vi "Parse Sentence_VTG.vi"(8 "error in (no error)":errorcluster, 11 "VTG sentence":string) -> (0 "error out":errorcluster, 3 "VTG  data":T1 {"type of fix"."mode" items=["Simulator", "Not Valid", "Estimated", "Differential", "Autonomous"]})   [LabVIEW 2024]
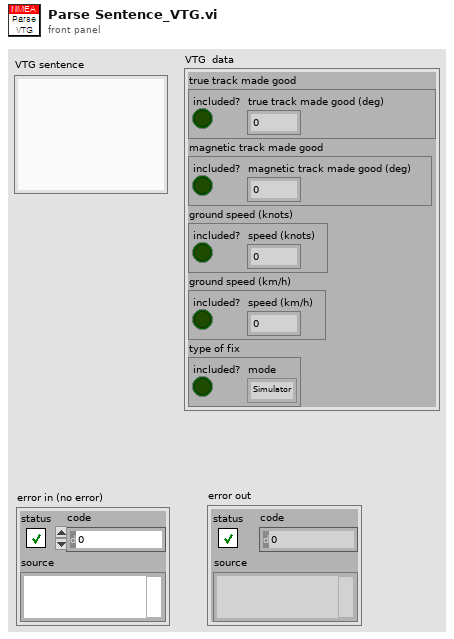
[diagram p1: front panel]
types:
  T1 = cluster{"true track made good":cluster{"included?":bool, "true track made good (deg)":dbl}, "magnetic track made good":cluster{"included?":bool, "magnetic track made good (deg)":dbl}, "ground speed (knots)":cluster{"included?":bool, "speed (knots)":dbl}, "ground speed (km/h)":cluster{"included?":bool, "speed (km/h)":dbl}, "type of fix":cluster{"included?":bool, "mode":u16}}
  T2 = cluster{"Boolean":bool, "True Track Made Good (Deg)":dbl}
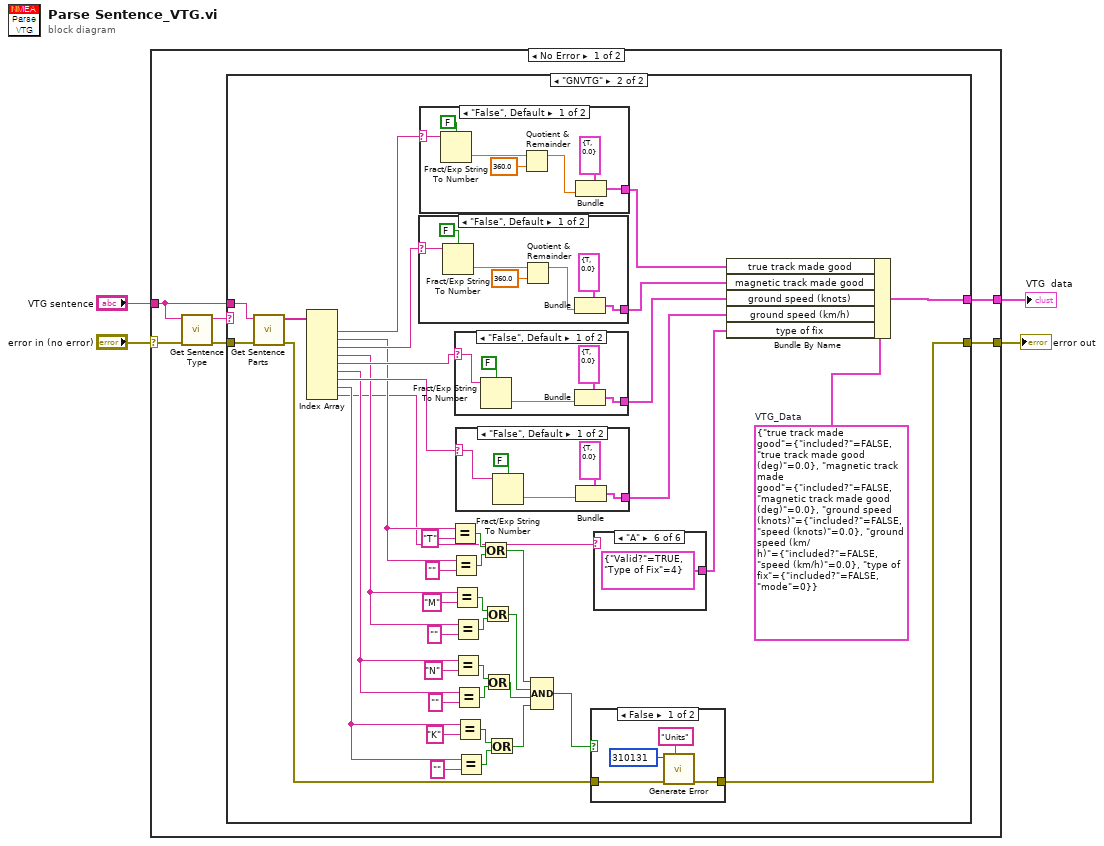
[diagram p0: block diagram]
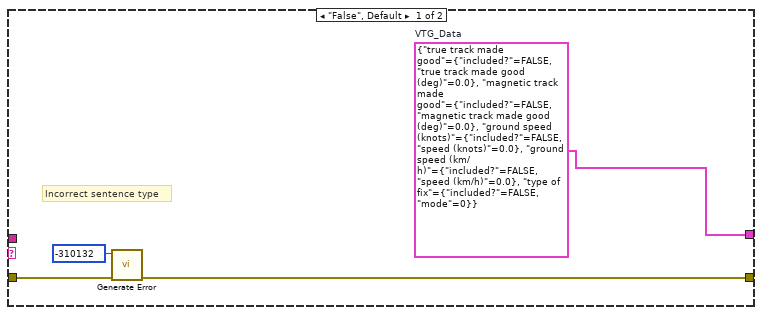
[diagram p2: hidden frame]
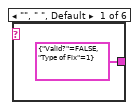
[diagram p3: hidden frame]
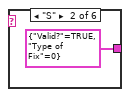
[diagram p4: hidden frame]
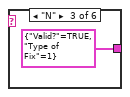
[diagram p5: hidden frame]
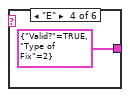
[diagram p6: hidden frame]
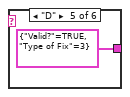
[diagram p7: hidden frame]
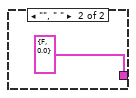
[diagram p9: hidden frame]
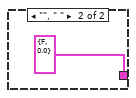
[diagram p10: hidden frame]
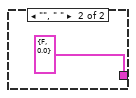
[diagram p11: hidden frame]
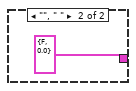
[diagram p12: hidden frame]
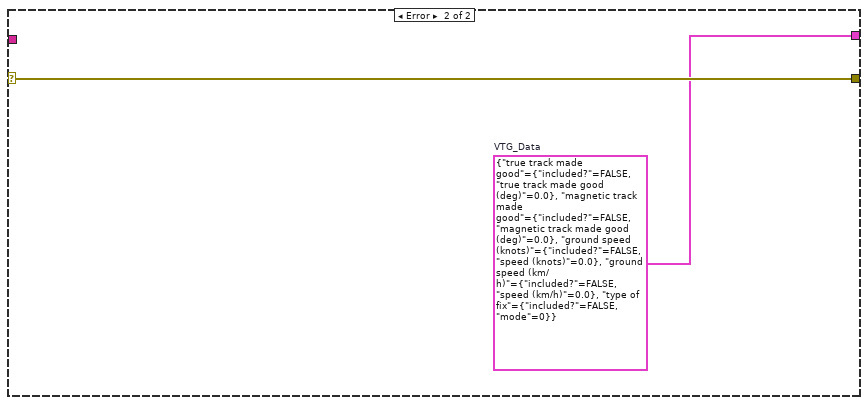
[diagram p13: hidden frame]
diagram:
  n1 = case shown="No Error" "error in (no error)" {
    selector: "error in (no error)" -> [w8 w97]
    tunnel: [w10 w96] -> w1
    tunnel: [w9 w97] -> w2
    tunnel: "VTG sentence" -> [w6 _]
    frame No Error {
      n2 = call "Get Sentence Type.vi"("error in (no error)"=w8, "sentence"=w6) -> ("error out"=w7:errorcluster, "sentence type"=w5:string)  [unwired: 7 in, 1 out]
      n3 = case shown="\"GNVTG\"" w5 {
        tunnel: w7 -> [w13 w56]
        tunnel: w6 -> [_ w19]
        tunnel: [w11 w55] -> w10
        tunnel: [w12 w16] -> w9
        frame "False", Default {
          w11 = T1 {"true track made good"={"included?"=FALSE, "true track made good (deg)"=0.0}, "magnetic track made good"={"included?"=FALSE, "magnetic track made good (deg)"=0.0}, "ground speed (knots)"={"included?"=FALSE, "speed (knots)"=0.0}, "ground speed (km/h)"={"included?"=FALSE, "speed (km/h)"=0.0}, "type of fix"={"included?"=FALSE, "mode"=0}}  # VTG_Data
          # "Incorrect sentence type"
          n4 = call "Generate Error.vi"("error in (no error)"=w13, "code"=-310132) -> ("error out"=w12:errorcluster)  [unwired: 9 in]
        }
        frame "GNVTG" {
          w15 = T1 {"true track made good"={"included?"=FALSE, "true track made good (deg)"=0.0}, "magnetic track made good"={"included?"=FALSE, "magnetic track made good (deg)"=0.0}, "ground speed (knots)"={"included?"=FALSE, "speed (knots)"=0.0}, "ground speed (km/h)"={"included?"=FALSE, "speed (km/h)"=0.0}, "type of fix"={"included?"=FALSE, "mode"=0}}  # VTG_Data
          n5 = call "Get Sentence Parts.vi"("error in (no error)"=w56, "sentence"=w19) -> ("error out"=w17:errorcluster, "sentence data"=w18:string[])  [unwired: 7 in, 1 out]
          n6 = Index Array(array=w18) -> (element #1=w53:string, element #2=w30:string, element #3=w47:string, element #4=w29:string, element #5=w48:string, element #6=w28:string, element #7=w49:string, element #8=w27:string, element #9=w21:string)  [unwired: 9 in]
          n7 = case shown="\"False\", Default" w47 {
            selector: w47 -> [w84 _]
            tunnel: [w85 T2 {"Boolean"=FALSE, "True Track Made Good (Deg)"=0.0} ("True Track Made Good")] -> w52
            frame "False", Default {
              n8 = Fract/Exp String To Number(use system decimal point (T)=FALSE, string=w84) -> (number=w83:dbl)  [unwired: 3 out]
              n9 = Quotient & Remainder(x=w83, y=360.0) -> (x-y*floor(x/y)=w82:dbl)  [unwired: 1 out]
              n10 = Bundle(cluster=T2 {"Boolean"=TRUE, "True Track Made Good (Deg)"=0.0} ("True Track Made Good"), "True Track Made Good (Deg)"=w82) -> (w85:T2)  [unwired: 1 out]
            }
            frame "", " " {
            }
          }
          n11 = case shown="\"False\", Default" w53 {
            selector: w53 -> [w92 _]
            tunnel: [w93 T2 {"Boolean"=FALSE, "True Track Made Good (Deg)"=0.0} ("True Track Made Good")] -> w54
            frame "False", Default {
              n12 = Fract/Exp String To Number(use system decimal point (T)=FALSE, string=w92) -> (number=w91:dbl)  [unwired: 3 out]
              n13 = Quotient & Remainder(x=w91, y=360.0) -> (x-y*floor(x/y)=w90:dbl)  [unwired: 1 out]
              n14 = Bundle(cluster=T2 {"Boolean"=TRUE, "True Track Made Good (Deg)"=0.0} ("True Track Made Good"), "True Track Made Good (Deg)"=w90) -> (w93:T2)  [unwired: 1 out]
            }
            frame "", " " {
            }
          }
          n15 = Equal?(x=w30, y="T") -> (x = y?=w45:bool)
          n16 = Equal?(x=w30, y="") -> (x = y?=w46:bool)
          n17 = Equal?(x=w29, y="M") -> (x = y?=w40:bool)
          n18 = Equal?(x=w29, y="") -> (x = y?=w39:bool)
          n19 = Equal?(x=w28, y="N") -> (x = y?=w32:bool)
          n20 = Equal?(x=w28, y="") -> (x = y?=w31:bool)
          n21 = case shown="\"False\", Default" w48 {
            selector: w48 -> [w75 _]
            tunnel: [w76 T2 {"Boolean"=FALSE, "True Track Made Good (Deg)"=0.0} ("True Track Made Good")] -> w51
            frame "False", Default {
              n22 = Fract/Exp String To Number(use system decimal point (T)=FALSE, string=w75) -> (number=w77:dbl)  [unwired: 3 out]
              n23 = Bundle(cluster=T2 {"Boolean"=TRUE, "True Track Made Good (Deg)"=0.0} ("True Track Made Good"), "True Track Made Good (Deg)"=w77) -> (w76:T2)  [unwired: 1 out]
            }
            frame "", " " {
            }
          }
          n24 = Equal?(x=w27, y="K") -> (x = y?=w37:bool)
          n25 = case shown="\"False\", Default" w49 {
            selector: w49 -> [w69 _]
            tunnel: [w70 T2 {"Boolean"=FALSE, "True Track Made Good (Deg)"=0.0} ("True Track Made Good")] -> w50
            frame "False", Default {
              n26 = Fract/Exp String To Number(use system decimal point (T)=FALSE, string=w69) -> (number=w71:dbl)  [unwired: 3 out]
              n27 = Bundle(cluster=T2 {"Boolean"=TRUE, "True Track Made Good (Deg)"=0.0} ("True Track Made Good"), "True Track Made Good (Deg)"=w71) -> (w70:T2)  [unwired: 1 out]
            }
            frame "", " " {
            }
          }
          n28 = Equal?(x=w27, y="") -> (x = y?=w38:bool)
          n29 = Or(x=w45, y=w46) -> (x .or. y?=w26:bool)
          n30 = Or(x=w40, y=w39) -> (x .or. y?=w23:bool)
          n31 = Or(x=w32, y=w31) -> (x .or. y?=w24:bool)
          n32 = Or(x=w37, y=w38) -> (x .or. y?=w25:bool)
          n33 = Compound Arithmetic op=AND(w26, w23, w24, w25) -> (w22:bool)
          n34 = case shown="False" w22 {
            tunnel: w17 -> [w64 w67]
            tunnel: [w63 w67] -> w16
            frame False {
              n35 = call "Generate Error.vi"("<append> (\"\")"="Units" ("<append> (\"\")"), "error in (no error)"=w64, "code"=310131) -> ("error out"=w63:errorcluster)  [unwired: 8 in]
            }
            frame True {
            }
          }
          n36 = case shown="\"A\"" w21 {
            tunnel: [cluster{"Valid?":bool, "Type of Fix":u16} {"Valid?"=FALSE, "Type of Fix"=1} ("Type of Fix") cluster{"Valid?":bool, "Type of Fix":u16} {"Valid?"=TRUE, "Type of Fix"=0} ("Type of Fix") cluster{"Valid?":bool, "Type of Fix":u16} {"Valid?"=TRUE, "Type of Fix"=1} ("Type of Fix") cluster{"Valid?":bool, "Type of Fix":u16} {"Valid?"=TRUE, "Type of Fix"=2} ("Type of Fix") cluster{"Valid?":bool, "Type of Fix":u16} {"Valid?"=TRUE, "Type of Fix"=3} ("Type of Fix") cluster{"Valid?":bool, "Type of Fix":u16} {"Valid?"=TRUE, "Type of Fix"=4} ("Type of Fix")] -> w20
            frame "", " ", Default {
            }
            frame "S" {
            }
            frame "N" {
            }
            frame "E" {
            }
            frame "D" {
            }
            frame "A" {
            }
          }
          n37 = Bundle By Name(cluster=w15, "true track made good"=w54, "magnetic track made good"=w52, "ground speed (knots)"=w51, "ground speed (km/h)"=w50, "type of fix"=w20) -> (w55:T1)
        }
      }
    }
    frame Error {
      w96 = T1 {"true track made good"={"included?"=FALSE, "true track made good (deg)"=0.0}, "magnetic track made good"={"included?"=FALSE, "magnetic track made good (deg)"=0.0}, "ground speed (knots)"={"included?"=FALSE, "speed (knots)"=0.0}, "ground speed (km/h)"={"included?"=FALSE, "speed (km/h)"=0.0}, "type of fix"={"included?"=FALSE, "mode"=0}}  # VTG_Data
    }
  }
  "error out" <- w2
  "VTG  data" <- w1
